vi "FPK_Control Property Set by Group.vi"(6 "FP Ctrl Aray":T2[](array[typedef]), 8 "Error":errorcluster, 9 "FP Ctrl Properies":T2, 10 "FP Group Array":T1[](array[typedef]), 11 "FP Control Group":T1) -> (0 "Error Out":errorcluster, 3 "Success Out":bool)   [LabVIEW 2020]
uses:
  TypeDefs_Utility/ENUM_FPK_Control Group Select.ctl
  TypeDefs_Utility/ENUM_FP_Hide Show Disable.ctl
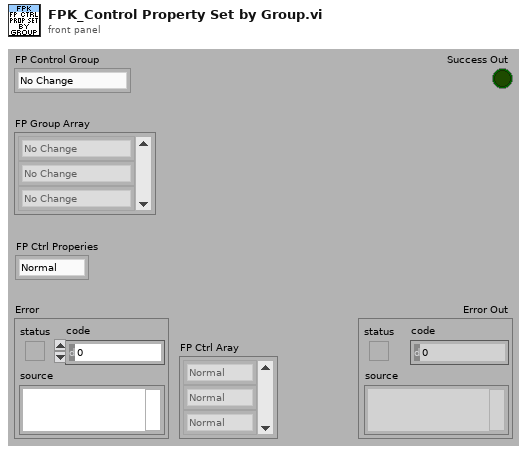
[diagram p1: front panel]
types:
  T1 = typedef "ENUM_FPK_Control Group Select.ctl" = enum16{"No Change", "ALL", "Manual; _M_", "Start; _S_", "SensorFrame; _SF_", "Information; _I_", "Plot; _P_"}
  T2 = typedef "ENUM_FP_Hide Show Disable.ctl" = enum16{"Normal", "Disable", "Disable Gray", "Hide"}
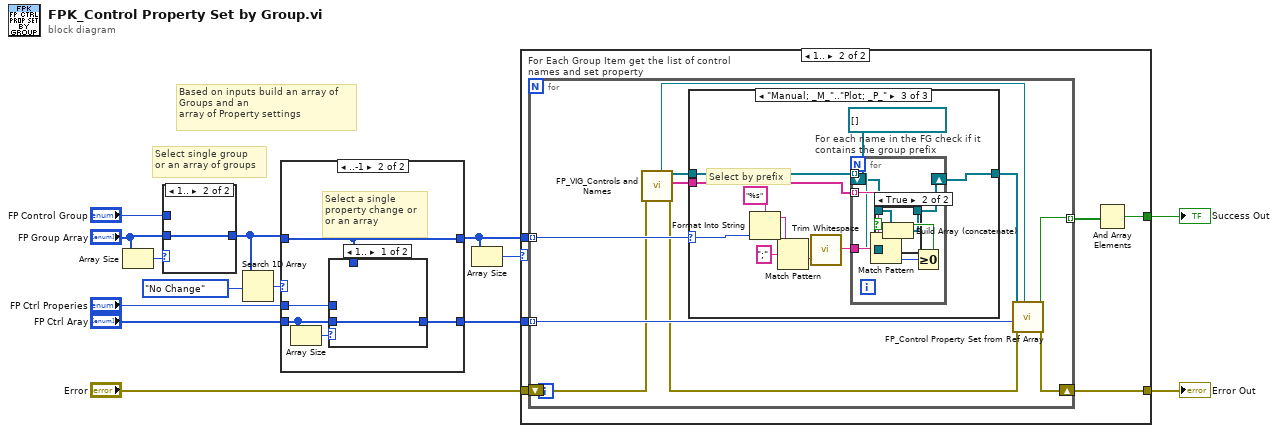
[diagram p0: block diagram]
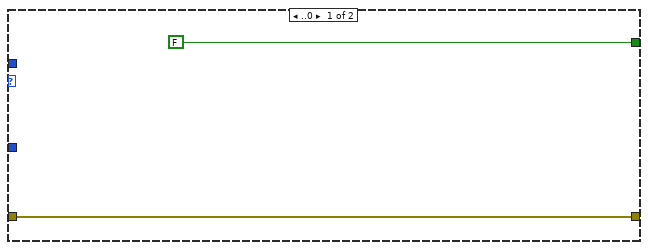
[diagram p2: hidden frame]
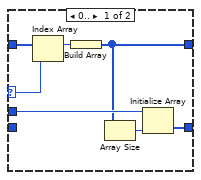
[diagram p6: hidden frame]
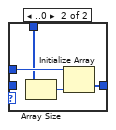
[diagram p7: hidden frame]
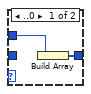
[diagram p8: hidden frame]
diagram:
  # "Select single group\nor an array of groups"
  # "Based on inputs build an array of \nGroups and an\narray of Property settings"
  n1 = Array Size(array="FP Group Array") -> (size(s)=w12:i32)
  n2 = case shown="1.." w12 {
    tunnel: "FP Group Array" -> [_ w17]
    tunnel: [w15 w17] -> w4
    tunnel: "FP Control Group" -> [w16 _]
    frame ..0 {
      n3 = Build Array(w16) -> (w15:T1[])
    }
    frame 1.. {
    }
  }
  n4 = Search 1D Array(1D array=w4, element=ENUM_FPK_Control_Group_Select."No Change") -> (index of element=w5:i32)  [unwired: 1 in]
  n5 = case shown="..-1" w5 {
    selector: w5 -> [w19 _]
    tunnel: "FP Ctrl Aray" -> [_ w26]
    tunnel: "FP Ctrl Properies" -> [w24 w29]
    tunnel: [w22 w28] -> w7
    tunnel: [w18 w27] -> w2
    tunnel: w4 -> [w21 w27]
    frame 0.. {
      n6 = Index Array(array=w21, index=w19) -> (element=w20:T1)
      n7 = Build Array(w20) -> (w18:T1[])
      n8 = Array Size(array=w18) -> (size(s)=w23:i32)
      n9 = Initialize Array(w24, w23) -> (w22:T2[])
    }
    frame ..-1 {
      # "Select a single\nproperty change or\nor an array"
      n10 = Array Size(array=w26) -> (size(s)=w25:i32)
      n11 = case shown="1.." w25 {
        tunnel: w29 -> [_ w34]
        tunnel: [w30 w32] -> w28
        tunnel: w27 -> [_ w31]
        tunnel: w26 -> [w30 _]
        frame 1.. {
        }
        frame ..0 {
          n12 = Array Size(array=w31) -> (size(s)=w33:i32)
          n13 = Initialize Array(w34, w33) -> (w32:T2[])
        }
      }
    }
  }
  n14 = Array Size(array=w2) -> (size(s)=w3:i32)
  n15 = case shown="1.." w3 {
    tunnel: "Error" -> [w35 w42]
    tunnel: [w35 w41] -> w14
    tunnel: [FALSE w39] -> w13
    tunnel: w7 -> [_ w38]
    tunnel: w2 -> [_ w37]
    frame ..0 {
    }
    frame 1.. {
      n16 = for "For Each Group Item get the list of control names and set property" {
        shift-right: [w48] -> w41
        shift-left: w42 -> [w44]
        tunnel: w37 -> [w52] mode=indexing
        tunnel: [w49] -> w40 mode=indexing
        tunnel: w38 -> [w50] mode=indexing
        n17 = call "FP_VIG_Controls and Names.vi"("Error"=w44) -> ("Error Out"=w43:errorcluster, "FP Names Out"=w45:string[], "FP Controls Out"=w46:refnum<vi>[], "FrontPanel Out"=w47:refnum<vi>)  [unwired: 7 in]
        n18 = case shown="\"Manual; _M_\"..\"Plot; _P_\"" w52 {
          selector: w52 -> [_ _ w62]
          tunnel: [_ _ w57] -> w51
          tunnel: w46 -> [_ _ w55]
          tunnel: w45 -> [_ _ w56]
          frame "No Change" {
          }
          frame "ALL" {
          }
          frame "Manual; _M_".."Plot; _P_" {
            # "Select by prefix"
            n19 = Format Into String(format string="%s", w62) -> (resulting string=w59:string)  [unwired: 2 in, 1 out]
            n20 = Match Pattern(string=w59, regular expression=";") -> (after substring=w58:string)  [unwired: 1 in, 3 out]
            n21 = call <vilib>:"Trim Whitespace.vi"("string"=w58) -> ("trimmed string"=w54:string)  [unwired: 1 in]
            n22 = for "For each name in the FG check if it\ncontains the group prefix" {
              tunnel: w56 -> [w68] mode=indexing
              tunnel: w54 -> [w69]
              tunnel: w55 -> [w66] mode=indexing
              shift-right: [w63] -> w57
              shift-left: refnum<vi>[] [] ("Array") -> [w64]
              n23 = Match Pattern(string=w68, regular expression=w69) -> (offset past match=w67:i32)  [unwired: 1 in, 3 out]
              n24 = Greater Or Equal To 0?(x=w67) -> (x >= 0?=w65:bool)
              n25 = case shown="True" w65 {
                tunnel: w64 -> [w70 w72]
                tunnel: w66 -> [_ w71]
                tunnel: [w70 w73] -> w63
                frame False {
                }
                frame True {
                  n26 = Build Array (concatenate)(w72, w71) -> (w73:refnum<vi>[])
                }
              }
            }
          }
        }
        n27 = call "FP_Control Property Set from Ref Array.vi"("Panel"=w47, "Error"=w43, "FP Ctrl Properies"=w50, "FP Controls"=w51) -> ("Error Out"=w48:errorcluster, "Success Out"=w49:bool)  [unwired: 6 in]
      }
      n28 = And Array Elements(Boolean array=w40) -> (logical AND=w39:bool)
    }
  }
  "Error Out" <- w14
  "Success Out" <- w13
